vi "Notebook Find String before.vi"(8 "error in (no error)":errorcluster, 9 "Before position":i32, 10 "Search String":string, 11 ".NET Refnum in":refnum<k24>) -> (0 "error out":errorcluster, 1 "Location after string":i32, 2 "String location":i32, 3 ".NET Refnum out":refnum<k24>)   [LabVIEW 2021, in "Notebook.lvlib"]
uses:
  Notebook.lvlib
  System.Windows.Forms
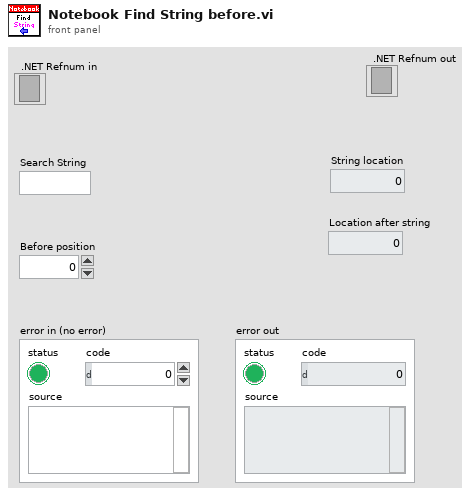
[diagram p1: front panel]
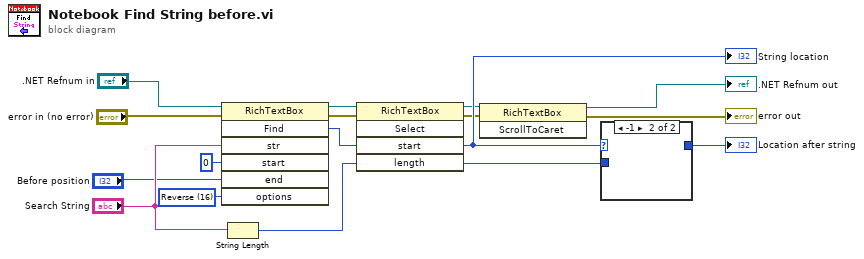
[diagram p0: block diagram]
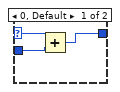
[diagram p2: hidden frame]
diagram:
  w3 = 16 items=["None"=0, "WholeWord"=2, "MatchCase"=4, "NoHighlight"=8, "Reverse"=16] ("options")
  n1 = invoke class="RichTextBox" method="Find"(reference=".NET Refnum in", error in="error in (no error)", "str"="Search String", "start"=0, "end"="Before position", "options"=w3) -> (reference out=w9:refnum<k24>, error out=w10:errorcluster, "Find"=w11:i32)  [unwired: 1 in, 4 out]
  "String location" <- w11
  n2 = String Length(string="Search String") -> (length=w15:i32)
  n3 = invoke class="RichTextBox" method="Select"(reference=w9, error in=w10, "start"=w11, "length"=w15) -> (reference out=w7:refnum<k24>, error out=w6:errorcluster)  [unwired: 1 in, 3 out]
  n4 = invoke class="RichTextBox" method="ScrollToCaret"(reference=w7, error in=w6) -> (reference out=→".NET Refnum out":refnum<k24>, error out=→"error out":errorcluster)  [unwired: 1 in, 1 out]
  n5 = case shown="-1" w11 {
    selector: w11 -> [w18 _]
    tunnel: [w17 _] -> w12
    tunnel: w15 -> [w16 _]
    frame 0, Default {
      n6 = Add(x=w18, y=w16) -> (x+y=w17:i32)
    }
    frame -1 {
    }
  }
  "Location after string" <- w12
